vi "类型3自动测试.vi"(10 "选择?":bool) -> ()   [LabVIEW 2010]
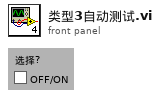
[diagram p1: front panel]
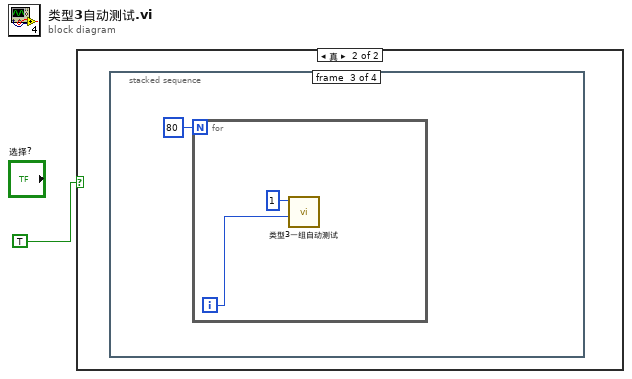
[diagram p0: block diagram]
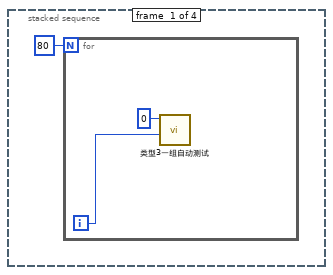
[diagram p3: hidden frame]
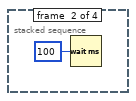
[diagram p4: hidden frame]
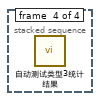
[diagram p5: hidden frame]
diagram:
  n1 = case shown="真" TRUE {
    frame False {
    }
    frame True {
      n2 = stacked-sequence {
        frame #0 {
          n3 = for {
            N: 80 -> [_]
            i -> [w3]
            n4 = call "类型3一组自动测试.vi"("第几个"=w3, "测试值"=0) -> ()  [unwired: 10 in]
          }
        }
        frame #1 {
          n5 = Wait (ms)(milliseconds to wait=u32 100 ("等待时间（毫秒）")) -> ()  [unwired: 1 out]
        }
        frame #2 {
          n6 = for {
            N: 80 -> [_]
            i -> [w7]
            n7 = call "类型3一组自动测试.vi"("第几个"=w7, "测试值"=1) -> ()  [unwired: 10 in]
          }
        }
        frame #3 {
          n8 = call "自动测试类型3统计结果.vi"() -> ()  [unwired: 12 in]
        }
      }
    }
  }
